vi "FPGA Configure FIFO.vi"(8 "error in (no error)":errorcluster, 9 "Depth":u64, 10 "FIFO":T1, 11 "FPGA Session In":refnum<class "Firmware Independent PID Interface.lvclass">) -> (0 "error out":errorcluster, 3 "FPGA Session Out":refnum<class "Firmware Independent PID Interface.lvclass">)   [LabVIEW 2010, in "Firmware Independent PID Interface.lvclass"]
doc: "Specifies the depth of the host memory part of the DMA FIFO. This method is optional."
uses:
  Firmware Independent PID Interface.lvclass
  TypeDefs/AllFifos.ctl
  <userlib>/_FPGA Interface Advanced Tools/FPGA Interface Base/FPGA Interface Base.lvclass/FPGA Interface Base.ctl
  <vilib>/Utility/error.llb/Error Cluster From Error Code.vi
  <userlib>/_FPGA Interface Advanced Tools/FPGA Interface Base/Accessors/FPGA Read Session.vi
  <userlib>/_FPGA Interface Advanced Tools/FPGA Interface Wrapper/FPGA Interface Wrapper.lvlib
  <userlib>/_FPGA Interface Advanced Tools/FPGA Interface Base/FPGA Interface Base.lvclass
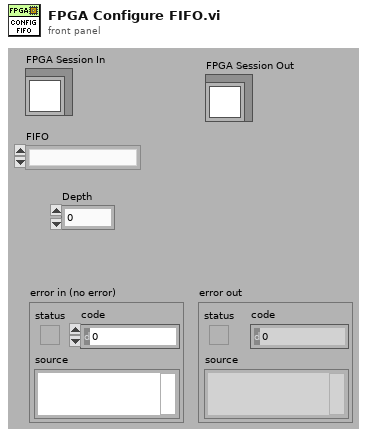
[diagram p1: front panel]
types:
  T1 = typedef "Firmware Independent PID Interface.lvclass/AllFifos.ctl" = enum16{""}
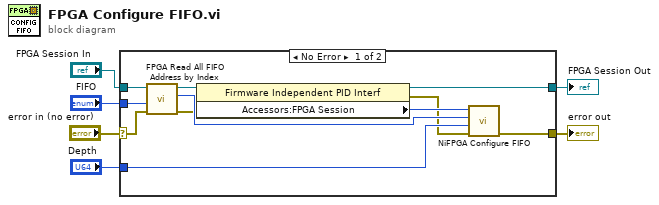
[diagram p0: block diagram]
diagram:
  n1 = case shown="No Error" "error in (no error)" {
    selector: "error in (no error)" -> [w15 w19]
    tunnel: [w7 w19] -> w2
    tunnel: [w8 w18] -> w1
    tunnel: "FPGA Session In" -> [w16 w18]
    tunnel: "FIFO" -> [w14 _]
    tunnel: "Depth" -> [w17 _]
    frame No Error {
      n2 = call <userlib>:"FPGA Read All FIFO Address by Index.vi"("error in (no error)"=w15, "index"=w14, "FPGA Interface Base in"=w16) -> ("error out"=w11:errorcluster, "Address"=w13:u32, "FPGA Interface Base out"=w12:refnum<class "Firmware Independent PID Interface.lvclass">)  [unwired: 5 in, 1 out]
      n3 = property class="Firmware Independent PID Interf"(reference=w12, error in=w11) -> (reference out=w8:refnum<class "Firmware Independent PID Interface.lvclass">, error out=w9:errorcluster, "Accessors:FPGA Session"=w10:u32)
      n4 = call <userlib>:"NiFPGA Configure FIFO.vi"("error in (no error)"=w9, "Depth"=w17, "FIFO"=w13, "Session"=w10) -> ("error out"=w7:errorcluster)  [unwired: 6 in, 1 out]
    }
    frame Error {
    }
  }
  "error out" <- w2
  "FPGA Session Out" <- w1
